vi "OAT Generate Error Cluster.vi"(1 "error in (no error)":errorcluster, 2 "Error Code":i32) -> (0 "error out":errorcluster)   [LabVIEW 2017]
doc: "Builds an error cluster with status set to True, code set to the Error Code control, and source set to the entire call chain down to the VI that called this."
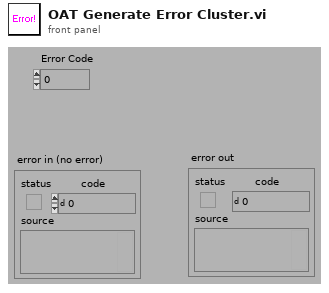
[diagram p1: front panel]
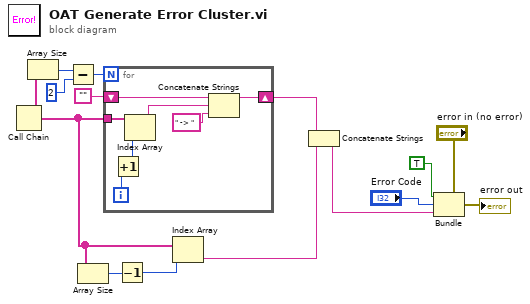
[diagram p0: block diagram]
diagram:
  n1 = Call Chain() -> (call chain=w6:string[])
  n2 = Array Size(array=w6) -> (size(s)=w9:i32)
  n3 = Subtract(x=w9, y=2) -> (x-y=w10:i32)
  n4 = Array Size(array=w6) -> (size(s)=w5:i32)
  n5 = for {
    N: w10 -> [_]
    tunnel: w6 -> [w19]
    shift-right: [w15] -> w3
    shift-left: "" -> [w18]
    i -> [w21]
    n6 = Increment(x=w21) -> (x+1=w20:i32)
    n7 = Index Array(array=w19, index=w20) -> (element=w17:string)
    n8 = Concatenate Strings(w18, w17, " -> " ("Substring")) -> (w15:string)
  }
  n9 = Decrement(x=w5) -> (x-1=w4:i32)
  n10 = Index Array(array=w6, index=w4) -> (element=w2:string)
  n11 = Concatenate Strings(w3, w2) -> (w1:string)
  n12 = Bundle(cluster="error in (no error)", "status"=TRUE ("Bundle Element"), "code"="Error Code", "source"=w1) -> (→"error out":errorcluster)
